vi "Create Callback.vi"(6 "Create Callback?":bool, 7 "Parent VI Ref":refnum<vi>, 9 "Template VI Ref":refnum<vi>, 11 "Callback Path":string) -> (1 "Saved Callback Path":path, 3 "Dup Callback Path":string)   [LabVIEW 2021]
uses:
  <vilib>/myRIO/Express VI/IRQ/Message Globals.vi
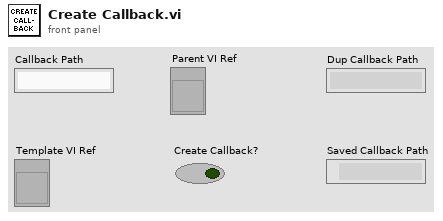
[diagram p1: front panel]
types:
  T1 = enum32{"invalid lock state", "Not Locked", "Locked (No Password)", "Password-protected"}
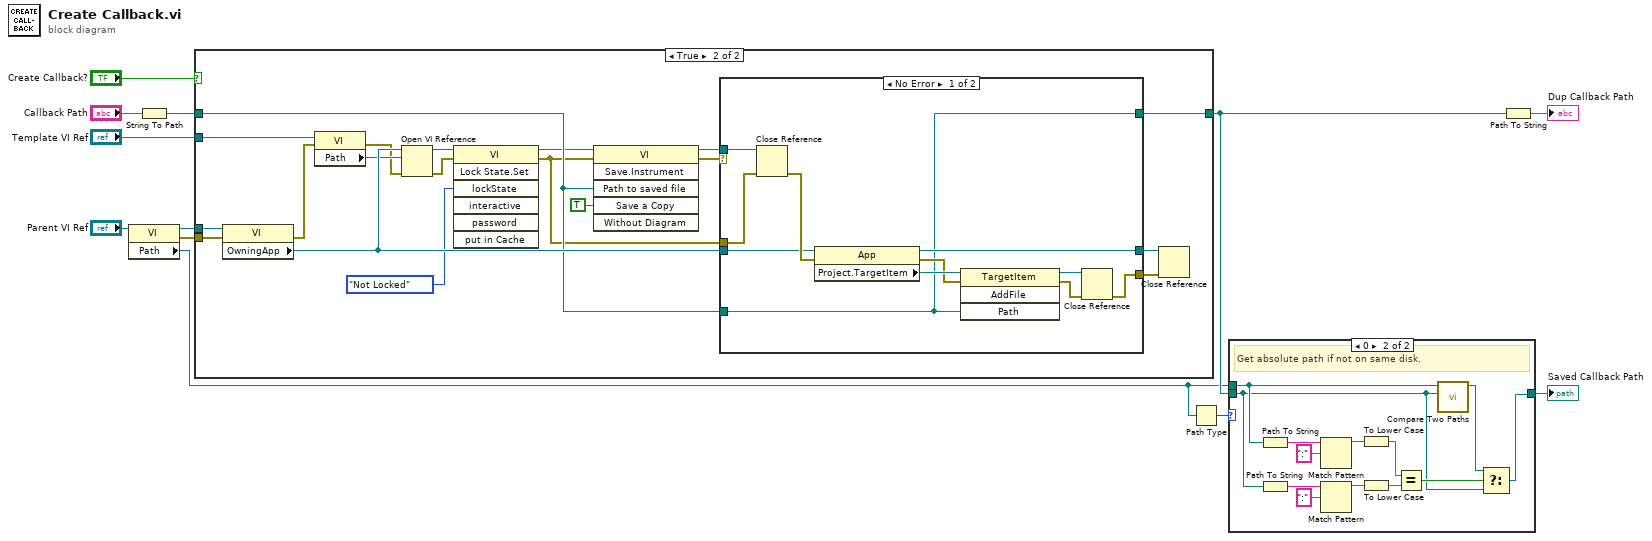
[diagram p0: block diagram]
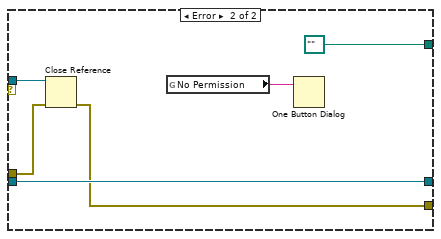
[diagram p4: hidden frame]
diagram:
  n1 = property class="VI"(reference="Parent VI Ref") -> (reference out=w8:refnum<vi>, error out=w7:errorcluster, "Path"=w3:path)  [unwired: 1 in]
  n2 = String To Path(string="Callback Path") -> (path=w5:path)
  n3 = case shown="True" "Create Callback?" {
    tunnel: "Template VI Ref" -> [_ w17]
    tunnel: w5 -> [w13 w22]
    tunnel: w8 -> [_ w31]
    tunnel: w7 -> [_ w23]
    tunnel: [w13 w24] -> w10
    frame False {
    }
    frame True {
      n4 = property class="VI"(reference=w31, error in=w23) -> (error out=w15:errorcluster, "OwningApp"=w27:refnum<vi>)  [unwired: 1 out]
      n5 = property class="VI"(reference=w17, error in=w15) -> (error out=w14:errorcluster, "Path"=w16:path)  [unwired: 1 out]
      n6 = Open VI Reference(application reference (local)=w27, vi path=w16, error in (no error)=w14) -> (vi reference=w26:refnum<vi>, error out=w20:errorcluster)  [unwired: 3 in]
      n7 = invoke class="VI" method="Lock State.Set"(reference=w26, error in=w20, "lockState"=T1."Not Locked" ("Lock State:Get")) -> (reference out=w21:refnum<vi>, error out=w19:errorcluster)  [unwired: 4 in, 5 out]
      n8 = invoke class="VI" method="Save.Instrument"(reference=w21, error in=w19, "Path to saved file"=w22, "Save a Copy"=TRUE) -> (reference out=w32:refnum<vi>, error out=w25:errorcluster)  [unwired: 2 in, 4 out]
      n9 = case shown="No Error" w25 {
        tunnel: w32 -> [w43 w49]
        tunnel: [w37 w47] -> w29
        tunnel: [w36 w46] -> w28
        tunnel: w27 -> [w35 w47]
        tunnel: w22 -> [w33 _]
        tunnel: w19 -> [w34 w48]
        tunnel: [w33 path "" ("dup path")] -> w24
        frame No Error {
          n10 = Close Reference(reference=w43, error in (no error)=w34) -> (error out=w41:errorcluster)
          n11 = property class="App"(reference=w35, error in=w41) -> (reference out=w37:refnum<vi>, error out=w40:errorcluster, "Project.TargetItem"=w42:refnum<vi>)
          n12 = invoke class="TargetItem" method="AddFile"(reference=w42, error in=w40, "Path"=w33) -> (reference out=w38:refnum<vi>, error out=w39:errorcluster)  [unwired: 1 in, 2 out]
          n13 = Close Reference(reference=w38, error in (no error)=w39) -> (error out=w36:errorcluster)
        }
        frame Error {
          n14 = Close Reference(reference=w49, error in (no error)=w48) -> (error out=w46:errorcluster)
          n15 = global read "Message Globals.vi" "No Permission"() -> (w45:string)
          n16 = One Button Dialog(message=w45) -> ()  [unwired: 1 in, 1 out]
        }
      }
      n17 = Close Reference(reference=w29, error in (no error)=w28) -> ()  [unwired: 1 out]
    }
  }
  n18 = Path Type(1:w3) -> (0:w2:i16)
  n19 = case shown="0" w2 {
    tunnel: w10 -> [w50 w52]
    tunnel: w3 -> [_ w63]
    tunnel: [w50 w51] -> w1
    frame Default {
      # "Get absolute path if owning VI not saved"
    }
    frame 0 {
      # "Get absolute path if not on same disk."
      n20 = Path To String(path=w63) -> (string=w61:string)
      n21 = Path To String(path=w52) -> (string=w59:string)
      n22 = Match Pattern(string=w61, regular expression=":") -> (before substring=w58:string)  [unwired: 1 in, 3 out]
      n23 = Match Pattern(string=w59, regular expression=":") -> (before substring=w57:string)  [unwired: 1 in, 3 out]
      n24 = To Lower Case(string=w58) -> (all lower case string=w56:string)
      n25 = To Lower Case(string=w57) -> (all lower case string=w55:string)
      n26 = Equal?(x=w56, y=w55) -> (x = y?=w54:bool)
      n27 = call <vilib>:"Compare Two Paths.vi"("Path 2"=w52, "Path 1"=w63) -> ("Relative Path from 1 to 2"=w53:path)  [unwired: 6 in, 3 out]
      n28 = Select(t=w53, s=w54, f=w52) -> (s? t:f=w51:path)
    }
  }
  "Saved Callback Path" <- w1
  n29 = Path To String(path=w10) -> (string=→"Dup Callback Path":string)
